vi "Read Roi_Filter.vi"(8 "error in (no error)":errorcluster, 11 "Sensor in":refnum<class "Sensor.lvclass">) -> (0 "error out":errorcluster, 2 "Roi_Filter":T1={"minAzimuth"=0.0, "maxAzimuth"=0.0, "minElevation"=0.0, "maxElevation"=0.0, "SiteA"=TRUE, "SiteB"=TRUE}, 3 "Sensor out":refnum<class "Sensor.lvclass">)   [LabVIEW 2018, in "Sensor.lvlib" / "Sensor.lvclass"]
uses:
  Sensor.lvclass
  Sensor.lvclass/Sensor.ctl
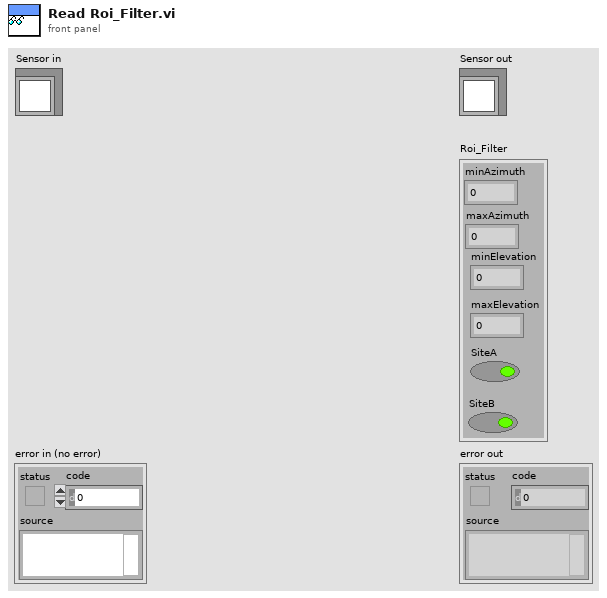
[diagram p1: front panel]
types:
  T1 = cluster{"minAzimuth":dbl, "maxAzimuth":dbl, "minElevation":dbl, "maxElevation":dbl, "SiteA":bool, "SiteB":bool}
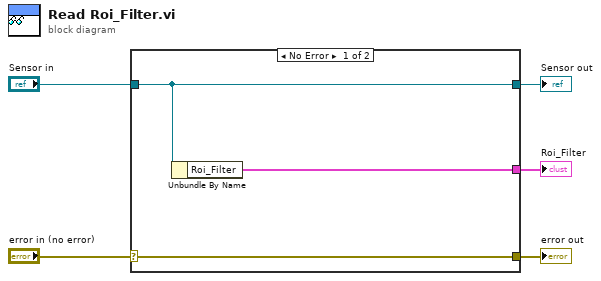
[diagram p0: block diagram]
diagram:
  n1 = case shown="No Error" "error in (no error)" {
    selector: "error in (no error)" -> [w8 w9]
    tunnel: [w8 w9] -> w4
    tunnel: [w7 w10] -> w2
    tunnel: "Sensor in" -> [w7 w10]
    tunnel: [w6 _] -> w1
    frame No Error {
      n2 = Unbundle By Name(w7) -> ("Roi_Filter"=w6:T1)
    }
    frame Error {
    }
  }
  "error out" <- w4
  "Sensor out" <- w2
  "Roi_Filter" <- w1
